vi "DT_Triangle Manager_Get Ghost Point.vi"(10 "triangle":i32, 11 "Triangles In":i32[][](array[numeric])) -> (2 "ghost point idx":i32)   [LabVIEW 2017, in "NI_AAL_Geometry.lvlib"]
uses:
  <vilib>/Analysis/NI_AAL_Geometry.lvlib
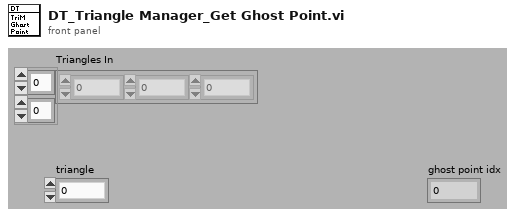
[diagram p1: front panel]
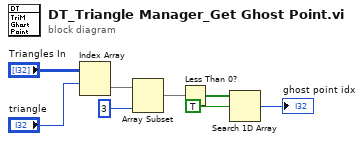
[diagram p0: block diagram]
diagram:
  n1 = Index Array(array="Triangles In", index (row)="triangle") -> (element=w2:i32[])  [unwired: 1 in]
  n2 = Array Subset(array=w2, length=3) -> (w5:i32[])  [unwired: 1 in]
  n3 = Less Than 0?(x=w5) -> (x < 0?=w4:bool[])
  n4 = Search 1D Array(1D array=w4, element=TRUE) -> (index of element=→"ghost point idx":i32)  [unwired: 1 out]
